vi "Read Average Power.vi"(8 "error in":errorcluster, 11 "2936r in":refnum<class "2936r.lvclass">) -> (0 "error out":errorcluster, 3 "2936r out":refnum<class "2936r.lvclass">)   [LabVIEW 2017, in "2936r.lvlib" / "2936r.lvclass"]
uses:
  2936r.lvclass
  2936r.lvclass/2936r.ctl
  Optical Power Meter.lvlibp/Optical Power Meter.lvclass
  C:/Users/Ron.Dexter.LUMINARTECH/Desktop/Power Meter/Optical Power Meter.lvlibp/Optical Power Meter.lvclass
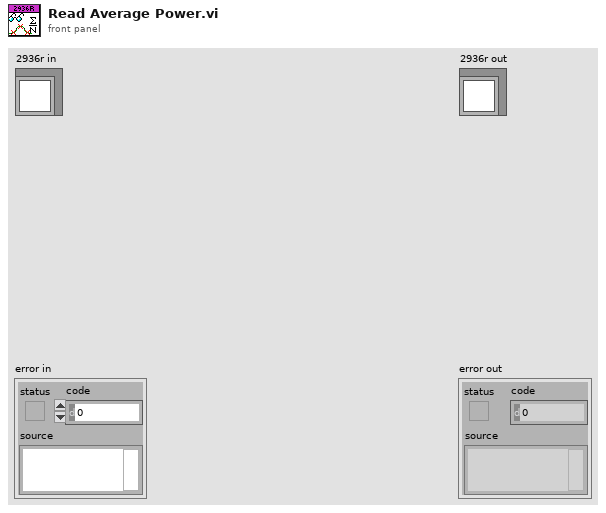
[diagram p1: front panel]
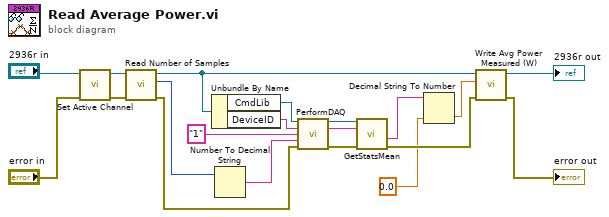
[diagram p0: block diagram]
diagram:
  n1 = call "Set Active Channel.vi"("error in (no error)"="error in", "2936r in"="2936r in") -> ("error out"=w17:errorcluster, "2936r out"=w18:refnum<class "2936r.lvclass">)  [unwired: 8 in]
  n2 = call "Read Number of Samples.vi"("error in (no error)"=w17, "Optical Power Meter in"=w18) -> ("error out"=w11:errorcluster, "Number of Samples"=w13:u64, "Optical Power Meter out"=w7:refnum<class "2936r.lvclass">)  [unwired: 7 in]
  n3 = Unbundle By Name(w7) -> ("CmdLib"=w16:refnum<k24>, "DeviceID"=w15:string)
  n4 = Number To Decimal String(number=w13) -> (decimal integer string=w12:string)  [unwired: 1 in]
  n5 = call <instrlib>:"PerformDAQ.vi"("PM Cmds In"=w16, "Device Key In"=w15, "Interval"="1", "Sample Size"=w12, "error in"=w11) -> ("PM Cmds Out"=w9:refnum<k24>, "Device Key Out"=w8:string, "error out"=w10:errorcluster)  [unwired: 7 in, 1 out]
  n6 = call <instrlib>:"GetStatsMean.vi"("error in"=w10, "Device Key In"=w8, "PM Cmds In"=w9) -> ("error out"=w3:errorcluster, "Mean"=w5:string)  [unwired: 5 in, 2 out]
  n7 = Decimal String To Number(string=w5, default (0L)=0.0) -> (number=w4:dbl)  [unwired: 1 in, 1 out]
  n8 = call "Write Avg Power Measured (W).vi"("error in (no error)"=w3, "Avg Power Measured (W)"=w4, "Optical Power Meter in"=w7) -> ("error out"=→"error out":errorcluster, "Optical Power Meter out"=→"2936r out":refnum<class "2936r.lvclass">)  [unwired: 7 in]
